vi "UI.vi"() -> (3 "Current File":path)   [LabVIEW 2020, in "FrameEditor.lvlib"]
doc: "This template is for the Queued Message Handler design pattern.\n\nThe Event Handling Loop generates messages based on user interface actions.\n\nThe Message Handling Loop processes messages generated by the Event Handling Loop, or by other messages. The messages are string values, so new messages can be added easily to the Message Cases case structure in the Message Handling Loop. Each message cluster can also provide an optional value for Message Data, which is a variant that can be converted to whatever message-specific data is required."
uses:
  FrameEditor.lvlib
  support/Message Queue/Message Queue.lvlib
  <vilib>/Utility/error.llb/Error Cluster From Error Code.vi
  support/User Event - Stop/User Event - Stop.lvlib
  support/Message Queue/Enqueue Message (Single).vi
  <vilib>/ErrorRing/Error Ring.xnode
  controls/UI Data.ctl
  Azdo/emea-aim-664-instrument-driver-1204/src/AIM664LV.lvlib
  controls/frame_record_type.ctl
  Azdo/emea-aim-664-instrument-driver-1204/src/_controls/queue_header_generic.ctl
  controls/frame_file_entry.ctl
  Azdo/emea-aim-664-instrument-driver-1204/src/_controls/queue_data_full.ctl
panel:
  in  "FrameID":string
  in  "Payload size":u32
  in  "Data":u8[](array[numeric])=[10] format="%.0x"
  in  "Frame Configuration":T1={"domainID"=1, "sideID"=1, "locationID"=1, "interfaceID"=1, "partitionID"=1} {"interfaceID" format="%.0b"}
  in  "VL Id":u16=60
  in  "UDPdstPort":u16=1
  in  "UDPsrcPort":u16=1
  in  "HeaderInfo":T2={"InterFrameGap"=0, "PacketGroupWaitTime"=10000, "PayloadBufferMode"=0, "PayloadGenerationMode"=0, "PreambleCount"=7, "Skew"=0, "NetSelect"=4, "FrameStartMode"=1, "PhysErrorInjection"=0, "SequenceNumberInit"=65535, "SequenceNumberOffset"=65535} {"NetSelect" items=["FDX_TX_FRAME_DLY_A"=0, "FDX_TX_FRAME_DLY_B"=1, "FDX_TX_FRAME_BOTH "=3, "FDX_TX_FRAME_ONLY_A"=4, "FDX_TX_FRAME_ONLY_B "=5]; "FrameStartMode" items=["FDX_TX_FRAME_START_IFG", "FDX_TX_FRAME_START_PGWT", "FDX_TX_FRAME_START_TRG"]; "PhysErrorInjection" items=["FDX_TX_FRAME_ERR_OFF"=0, "FDX_TX_FRAME_ERR_CRC"=1, "FDX_TX_FRAME_ERR_ALI"=2, "FDX_TX_FRAME_ERR_PRE"=4, "FDX_TX_FRAME_ERR_PHY"=8]; "SequenceNumberInit" items=["FDX_TX_FRAME_SEQ_INIT_AUTO"=65535]; "SequenceNumberOffset" items=["FDX_TX_FRAME_SEQ_OFFS_AUTO "=65535]; "PayloadGenerationMode" items=["FDX_TX_FRAME_PGM_USER"=0, "FDX_TX_FRAME_PGM_IP_PART"=1, "FDX_TX_FRAME_PGM_IP_FULL"=2, "FDX_TX_FRAME_PGM_IP_PART_TT"=10, "FDX_TX_FRAME_PGM_IP_FULL_TT"=20]; "PayloadBufferMode" items=["FDX_TX_FRAME_PBM_STD", "FDX_TX_FRAME_PBM_MAC", "FDX_TX_FRAME_PBM_UDP"]}
  in  "Load":bool
  in  "Save":bool
  in  "Frames":i32(listbox)
  out "Display <Replace Me>":string
  in  "Remove":bool
  in  "Add":bool
  in  "Exit":bool
  # "add new"
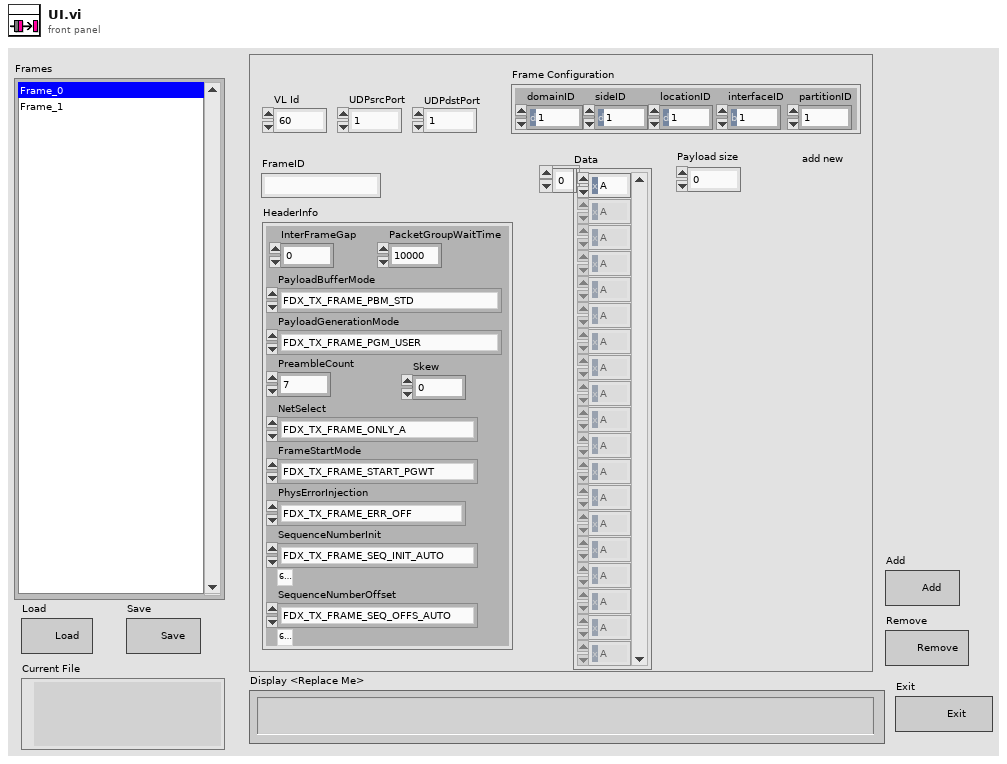
[diagram p1: front panel]
types:
  T1 = typedef "AIM664LV.lvlib/queue_data_full.ctl" = cluster{"domainID":u8, "sideID":u8, "locationID":u8, "interfaceID":u8, "partitionID":u8}
  T2 = typedef "AIM664LV.lvlib/queue_header_generic.ctl" = cluster{"InterFrameGap":u32, "PacketGroupWaitTime":u32, "PayloadBufferMode":u8, "PayloadGenerationMode":u8, "PreambleCount":u8, "Skew":u32, "NetSelect":u8, "FrameStartMode":u8, "PhysErrorInjection":u32, "SequenceNumberInit":u16, "SequenceNumberOffset":u16}
  T3 = typedef "FrameEditor.lvlib/frame_record_type.ctl" = cluster{"HeaderInfo":T2, "Data":u8[]}
  T4 = typedef "FrameEditor.lvlib/UI Data.ctl" = cluster{"Boolean <Replace Me>":bool, "String <Replace Me>":string, "Numeric <Replace Me>":dbl, "Add":refnum<vi>, "Remove":refnum<vi>, "Data Display Ref":refnum<vi>, "Exit Button Ref":refnum<vi>, "Load":refnum<vi>, "Save":refnum<vi>}
  T5 = typedef "FrameEditor.lvlib/Message Queue.lvlib/All Message Queues.ctl" = cluster{"UI":refnum<queue>}
  T6 = typedef "FrameEditor.lvlib/frame_file_entry.ctl" = cluster{"key":string, "value":T3}
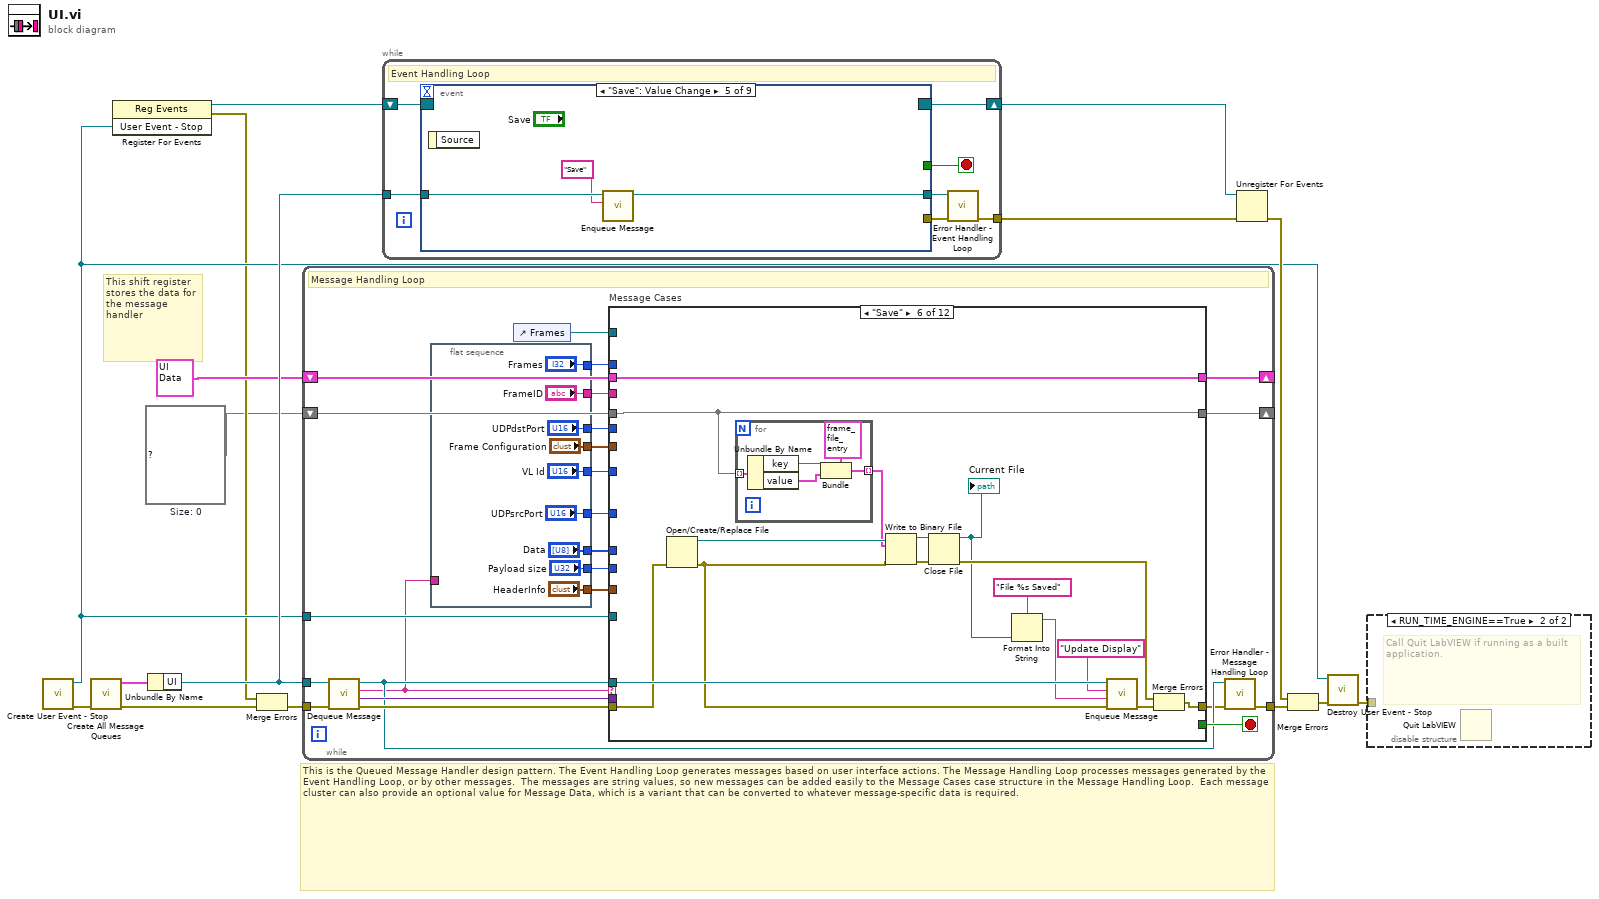
[diagram p0: block diagram]
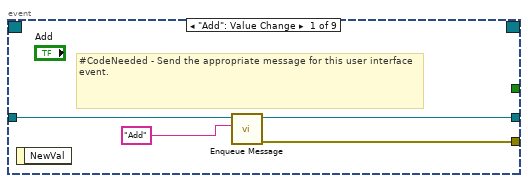
[diagram p3: hidden frame]
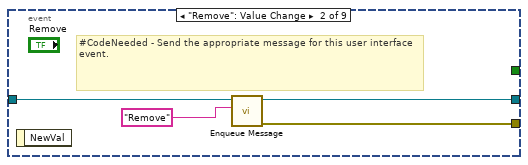
[diagram p4: hidden frame]
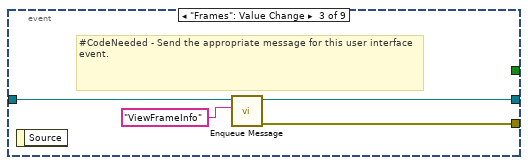
[diagram p5: hidden frame]
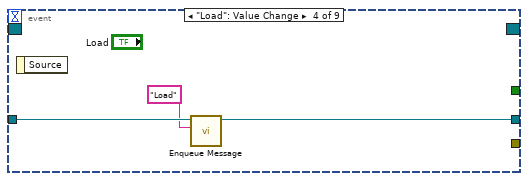
[diagram p6: hidden frame]
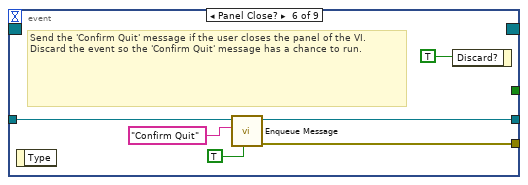
[diagram p7: hidden frame]
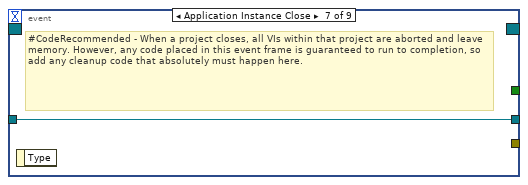
[diagram p8: hidden frame]
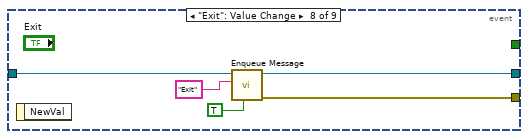
[diagram p9: hidden frame]
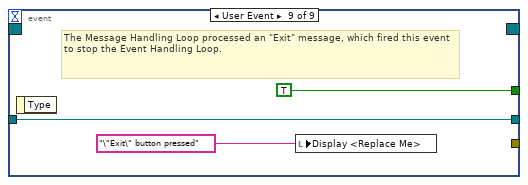
[diagram p10: hidden frame]
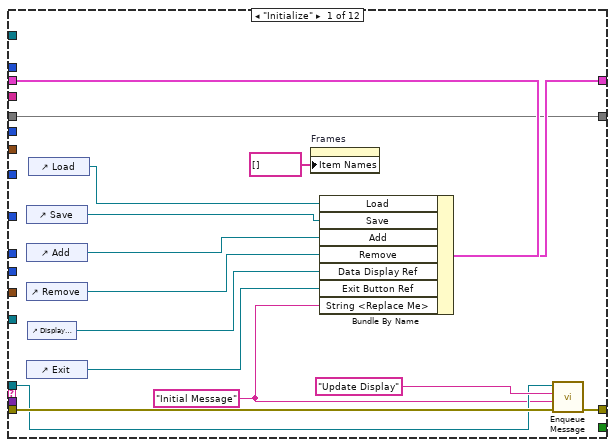
[diagram p11: hidden frame]
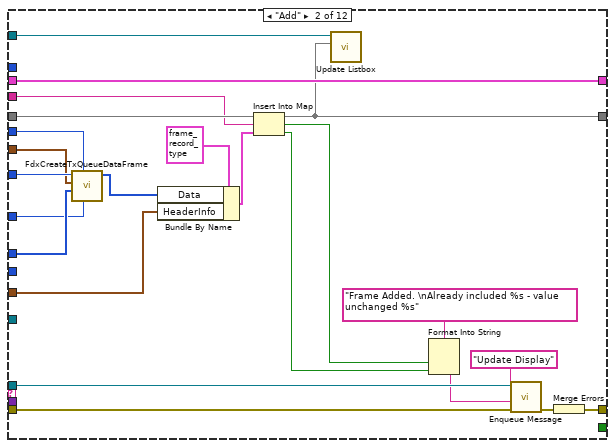
[diagram p12: hidden frame]
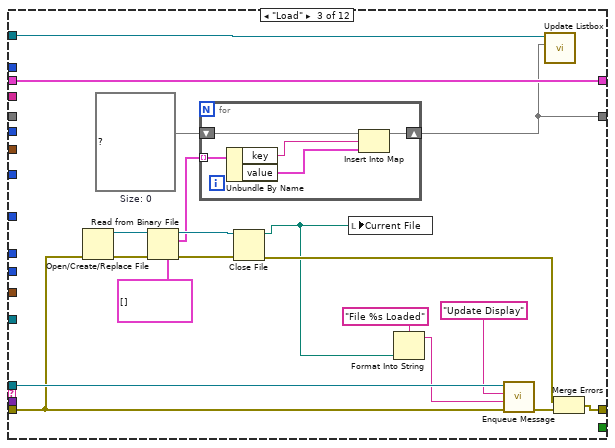
[diagram p13: hidden frame]
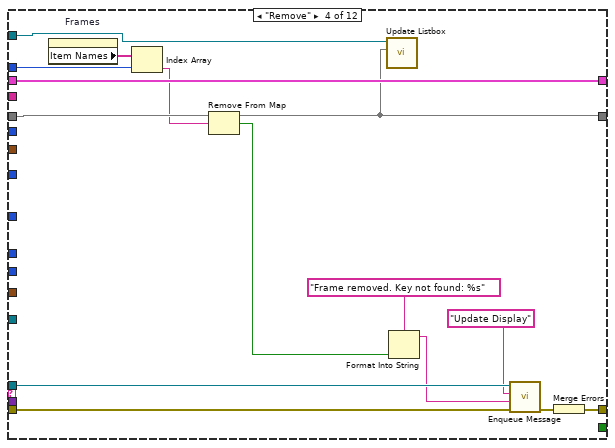
[diagram p14: hidden frame]
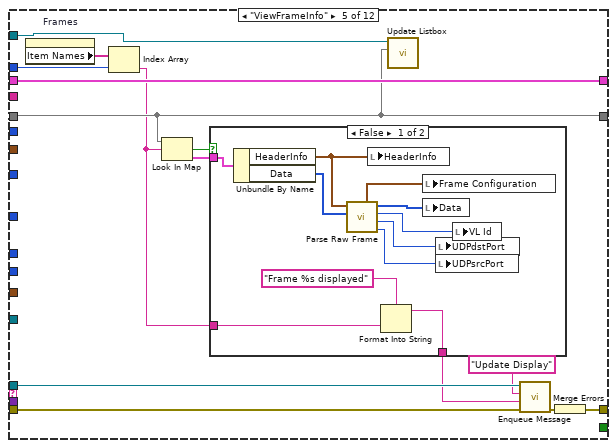
[diagram p15: hidden frame]
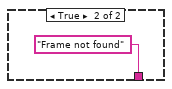
[diagram p16: hidden frame]
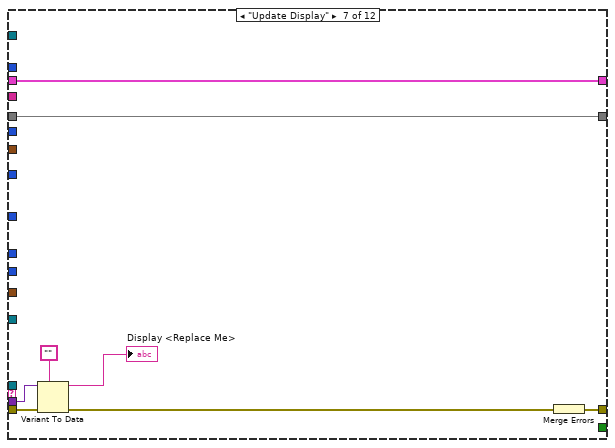
[diagram p17: hidden frame]
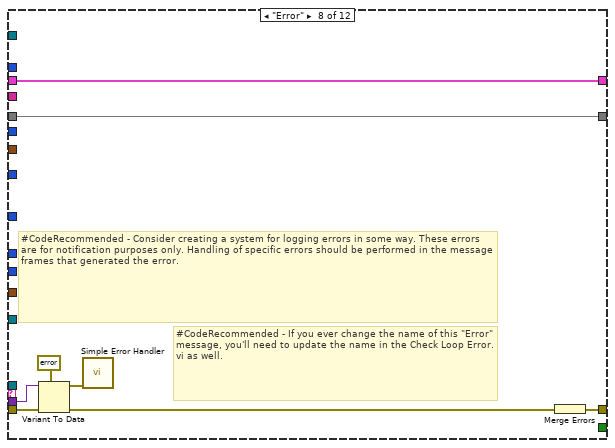
[diagram p18: hidden frame]
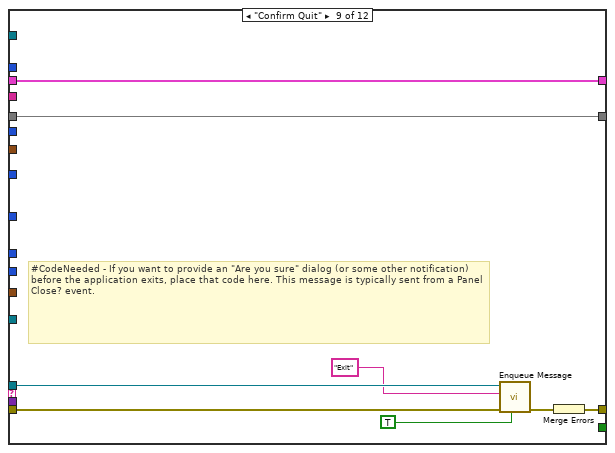
[diagram p19: hidden frame]
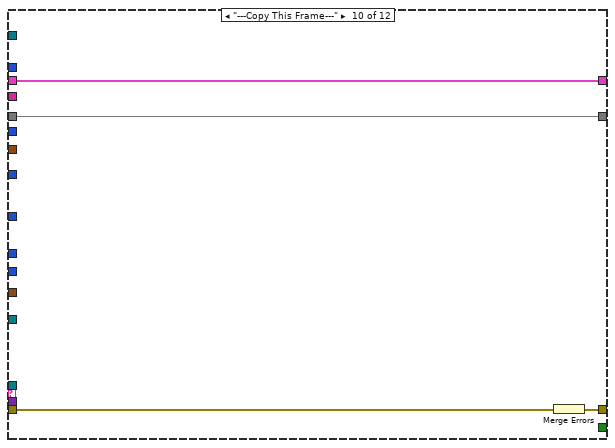
[diagram p20: hidden frame]
diagram:
  w1 = map{string, T3} {}  # Size: 0
  # "This is the Queued Message Handler design pattern. The Event Handling Loop generates messages based on user interface actions. The Message Handling Loop processes messages generated by the Event Handling Loop, or by other messages.  The messages are string values, so new messages can be added easily to the Message Cases case structure in the Message Handling Loop.  Each message cluster can also provide an optional value for Message Data, which is a variant that can be converted to whatever message-specific data is required."
  # "This shift register stores the data for the message handler"
  n1 = call "Create User Event - Stop.vi"() -> ("error out"=w12:errorcluster, "User Event - Stop"=w4:refnum<user-event>)  [unwired: 10 in]
  n2 = call "Create All Message Queues.vi"("error in (no error)"=w12) -> ("error out"=w16:errorcluster, "Message Queues out"=w15:T5)  [unwired: 9 in]
  n3 = register-events(w4) -> (reference out=w5:refnum<event-registration>, error out=w2:errorcluster)  [unwired: 2 in]
  n4 = Unbundle By Name(w15) -> ("UI"=w13:refnum<queue>)
  n5 = Merge Errors(w2, w16) -> (w3:errorcluster)
  n6 = while {
    tunnel: w13 -> [w33]
    shift-right: [w39] -> _
    shift-left: T4 {"Boolean <Replace Me>"=FALSE, "String <Replace Me>"="", "Numeric <Replace Me>"=0.0, "Add"=refnum, "Remove"=refnum, "Data Display Ref"=refnum, "Exit Button Ref"=refnum, "Load"=refnum, "Save"=refnum} ("Data Cluster") -> [w40]
    tunnel: w4 -> [w37]
    tunnel: w3 -> [w36]
    tunnel: [w31] -> w14
    shift-right: [w20] -> _
    shift-left: w1 -> [w22]
    stop <- w38 stop-if-true
    # "Message Handling Loop"
    n7 = call "Dequeue Message.vi"("error in (no error)"=w36, "Message Queue"=w33) -> ("error out"=w35:errorcluster, "Message Data"=w34:variant, "Message"=w17:string, "dup Message Queue"=w32:refnum<queue>)  [unwired: 6 in]
    n8 = flat-sequence {
      tunnel: ["Payload size"] -> w29
      tunnel: ["Frame Configuration"] -> w28
      tunnel: ["VL Id"] -> w27
      tunnel: ["UDPsrcPort"] -> w26
      tunnel: ["UDPdstPort"] -> w25
      tunnel: ["Data"] -> w24
      tunnel: ["HeaderInfo"] -> w23
      tunnel: ["FrameID"] -> w21
      tunnel: ["Frames"] -> w19
      tunnel: w17 -> [_]
      frame #0 {
      }
    }
    n9 = control-ref of="Frames"() -> (w18:refnum<vi>)
    n10 = case "Message Cases" shown="\"Save\"" w17 {
      selector: w17 -> [_ _ _ _ _ _ _ _ _ _ _ w215]
      tunnel: w32 -> [w55 w83 w103 w122 w136 w165 _ _ w193 _ w213 _]
      tunnel: w35 -> [w63 w85 w100 w124 w138 w163 w179 w189 w197 w201 w206 _]
      tunnel: [w64 w86 w105 w125 w139 w167 w180 w183 w195 w199 w209 w216] -> w30
      tunnel: w40 -> [w62 w87 w106 w126 w140 w168 w181 w188 w196 w200 w212 w217]
      tunnel: [w61 w87 w106 w126 w140 w168 w181 w188 w196 w200 w212 w217] -> w39
      tunnel: [_ _ _ _ _ _ _ _ _ _ TRUE _] -> w38
      tunnel: w34 -> [_ _ _ _ _ _ w178 w187 _ _ w203 _]
      tunnel: w37 -> [_ _ _ _ _ _ _ _ _ _ w208 _]
      tunnel: w29 -> [_ _ _ _ _ _ _ _ _ _ _ _]
      tunnel: w28 -> [_ w80 _ _ _ _ _ _ _ _ _ _]
      tunnel: w27 -> [_ w81 _ _ _ _ _ _ _ _ _ _]
      tunnel: w26 -> [_ w77 _ _ _ _ _ _ _ _ _ _]
      tunnel: w25 -> [_ w79 _ _ _ _ _ _ _ _ _ _]
      tunnel: w24 -> [_ w78 _ _ _ _ _ _ _ _ _ _]
      tunnel: w23 -> [_ w72 _ _ _ _ _ _ _ _ _ _]
      tunnel: w22 -> [w51 w76 _ w118 w132 w162 w174 w182 w190 w198 w202 w214]
      tunnel: w21 -> [_ w75 _ _ _ _ _ _ _ _ _ _]
      tunnel: [w51 w69 w91 w115 w132 w162 w174 w182 w190 w198 w202 w214] -> w20
      tunnel: w19 -> [_ _ _ w119 w134 _ _ _ _ _ _ _]
      tunnel: w18 -> [_ w70 w101 w116 w133 _ _ _ _ _ _ _]
      frame "Initialize" {
        w54 = "Initial Message" ("Initial Message")
        # "Initialize - All initialization work should take place in this message, since other loops can potentially enqueue messages that execute immediately after this one."
        n11 = control-ref of="Save"() -> (w52:refnum<vi>)
        n12 = control-ref of="Add"() -> (w60:refnum<vi>)
        n13 = control-ref of="Remove"() -> (w59:refnum<vi>)
        n14 = control-ref of="Exit"() -> (w57:refnum<vi>)
        n15 = control-ref of="Display <Replace Me>"() -> (w58:refnum<vi>)
        n16 = control-ref of="Load"() -> (w53:refnum<vi>)
        n17 = property on="Frames" class="LstBox (strict)"("Item Names"=string[] []) -> ()  [unwired: 2 in, 2 out]
        n18 = Bundle By Name(cluster=w62, "Load"=w53, "Save"=w52, "Add"=w60, "Remove"=w59, "Data Display Ref"=w58, "Exit Button Ref"=w57, "String <Replace Me>"=w54) -> (w61:T4)
        n19 = call-poly "Enqueue Message.vi"("error in (no error)"=w63, "Message Data"=w54, "Message"="Update Display", "Message Queue"=w55) -> ("error out"=w64:errorcluster)  [unwired: 6 in, 1 out]
      }
      frame "Add" {
        # "Something - Replace this message with functionality for your own application."
        n20 = call "FdxCreateTxQueueDataFrame.vi"("UDPsrcPort"=w77, "UDPdstPort"=w79, "Payload"=w78, "afdx configuration"=w80, "VL Id"=w81) -> ("Frame"=w71:u8[])  [unwired: 4 in, 2 out]
        n21 = Bundle By Name(cluster=T3 {"HeaderInfo"={"InterFrameGap"=0, "PacketGroupWaitTime"=10000, "PayloadBufferMode"=0, "PayloadGenerationMode"=0, "PreambleCount"=7, "Skew"=0, "NetSelect"=4, "FrameStartMode"=1, "PhysErrorInjection"=0, "SequenceNumberInit"=65535, "SequenceNumberOffset"=65535}, "Data"=[10]}, "Data"=w71, "HeaderInfo"=w72) -> (w73:T3)
        n22 = Insert Into Map(map in=w76, key=w75, value=w73) -> (map out=w69:map{string, T3}, key already included?=w66:bool, value unchanged?=w65:bool)
        n23 = call "Update Listbox.vi"("frame map"=w69, "ListBox ref"=w70) -> ()  [unwired: 10 in]
        n24 = Format Into String(format string="Frame Added. \nAlready included %s - value unchanged %s", w66, w65) -> (resulting string=w67:string)  [unwired: 2 in, 1 out]
        n25 = call-poly "Enqueue Message.vi"("error in (no error)"=w85, "Message Data"=w67, "Message"="Update Display", "Message Queue"=w83) -> ("error out"=w84:errorcluster)  [unwired: 6 in, 1 out]
        n26 = Merge Errors(w84) -> (w86:errorcluster)
      }
      frame "Load" {
        w93 = map{string, T3} {}  # Size: 0
        # "Something - Replace this message with functionality for your own application."
        n27 = Open/Create/Replace File(error in=w100) -> (refnum out=w95:refnum<file>, error out=w99:errorcluster)  [unwired: 5 in, 1 out]
        n28 = Read from Binary File(5:T6[] [] ("cluster"), 8:w99, 11:w95) -> (0:w98:errorcluster, 2:w92:T6[], 3:w96:refnum<file>)  [unwired: 3 in, 1 out]
        n29 = for {
          shift-right: [w110] -> w91
          shift-left: w93 -> [w111]
          tunnel: w92 -> [w109] mode=indexing
          n30 = Unbundle By Name(w109) -> ("key"=w108:string, "value"=w107:T3)
          n31 = Insert Into Map(map in=w111, key=w108, value=w107) -> (map out=w110:map{string, T3})  [unwired: 2 out]
        }
        n32 = Close File(refnum=w96, error in=w98) -> (path=w88:path, error out=w97:errorcluster)
        n33 = local write "Current File"(w88) -> ()
        n34 = Format Into String(format string="File %s Loaded", w88) -> (resulting string=w89:string)  [unwired: 2 in, 1 out]
        n35 = call-poly "Enqueue Message.vi"("error in (no error)"=w100, "Message Data"=w89, "Message"="Update Display", "Message Queue"=w103) -> ("error out"=w104:errorcluster)  [unwired: 6 in, 1 out]
        n36 = call "Update Listbox.vi"("frame map"=w91, "ListBox ref"=w101) -> ()  [unwired: 10 in]
        n37 = Merge Errors(w97, w104) -> (w105:errorcluster)
      }
      frame "Remove" {
        # "Something Else - Replace this message with functionality for your own application."
        n38 = property on="Frames" class="LstBox (strict)"() -> ("Item Names"=w120:string[])  [unwired: 2 in, 2 out]
        n39 = Index Array(array=w120, index=w119) -> (element=w117:string)
        n40 = Remove From Map(10:w117, 11:w118) -> (2:w112:bool, 3:w115:map{string, T3})  [unwired: 1 out]
        n41 = call "Update Listbox.vi"("frame map"=w115, "ListBox ref"=w116) -> ()  [unwired: 10 in]
        n42 = Format Into String(format string="Frame removed. Key not found: %s", w112) -> (resulting string=w113:string)  [unwired: 2 in, 1 out]
        n43 = call-poly "Enqueue Message.vi"("error in (no error)"=w124, "Message Data"=w113, "Message"="Update Display", "Message Queue"=w122) -> ("error out"=w123:errorcluster)  [unwired: 6 in, 1 out]
        n44 = Merge Errors(w123) -> (w125:errorcluster)
      }
      frame "ViewFrameInfo" {
        # "Something Else - Replace this message with functionality for your own application."
        n45 = property on="Frames" class="LstBox (strict)"() -> ("Item Names"=w135:string[])  [unwired: 2 in, 2 out]
        n46 = Index Array(array=w135, index=w134) -> (element=w127:string)
        n47 = Look In Map(map=w132, key=w127) -> (key not found?=w131:bool, value=w130:T3)  [unwired: 1 in]
        n48 = case shown="False" w131 {
          tunnel: w130 -> [w151 _]
          tunnel: [w148 "Frame not found"] -> w128
          tunnel: w127 -> [w149 _]
          frame False {
            n49 = Unbundle By Name(w151) -> ("HeaderInfo"=w147:T2, "Data"=w144:u8[])
            n50 = call "Parse Raw Frame.vi"("Data"=w144, "HeaderInfo"=w147) -> ("UDPsrcPort"=w141:u16, "UDPdstPort"=w142:u16, "VL Id"=w143:u16, "Payload"=w146:u8[], "Frame Configuration"=w145:T1)  [unwired: 5 in]
            n51 = local write "HeaderInfo"(w147) -> ()
            n52 = Format Into String(format string="Frame %s displayed", w149) -> (resulting string=w148:string)  [unwired: 2 in, 1 out]
            n53 = local write "Frame Configuration"(w145) -> ()
            n54 = local write "Data"(w146) -> ()
            n55 = local write "UDPdstPort"(w142) -> ()
            n56 = local write "UDPsrcPort"(w141) -> ()
            n57 = local write "VL Id"(w143) -> ()
          }
          frame True {
          }
        }
        n58 = call "Update Listbox.vi"("frame map"=w132, "ListBox ref"=w133) -> ()  [unwired: 10 in]
        n59 = call-poly "Enqueue Message.vi"("error in (no error)"=w138, "Message Data"=w128, "Message"="Update Display", "Message Queue"=w136) -> ("error out"=w137:errorcluster)  [unwired: 6 in, 1 out]
        n60 = Merge Errors(w137) -> (w139:errorcluster)
      }
      frame "Save" {
        # "Something Else - Replace this message with functionality for your own application."
        n61 = Open/Create/Replace File(error in=w163) -> (refnum out=w161:refnum<file>, error out=w160:errorcluster)  [unwired: 5 in, 1 out]
        n62 = for {
          tunnel: w162 -> [w173] mode=indexing
          tunnel: [w170] -> w156 mode=indexing
          n63 = Unbundle By Name(w173) -> ("key"=w172:string, "value"=w171:T3)
          n64 = Bundle(cluster=T6 {"key"="", "value"={"HeaderInfo"={"InterFrameGap"=0, "PacketGroupWaitTime"=0, "PayloadBufferMode"=0, "PayloadGenerationMode"=0, "PreambleCount"=0, "Skew"=0, "NetSelect"=0, "FrameStartMode"=0, "PhysErrorInjection"=0, "SequenceNumberInit"=0, "SequenceNumberOffset"=0}, "Data"=[]}}, "key"=w172, "value"=w171) -> (w170:T6)
        }
        n65 = Write to Binary File(file (use dialog)=w161, data=w156, error in=w160) -> (refnum out=w158:refnum<file>, error out=w159:errorcluster)  [unwired: 3 in, 1 out]
        n66 = Close File(refnum=w158, error in=w159) -> (path=w153:path, error out=w157:errorcluster)
        "Current File" <- w153
        n67 = Format Into String(format string="File %s Saved", w153) -> (resulting string=w155:string)  [unwired: 2 in, 1 out]
        n68 = call-poly "Enqueue Message.vi"("error in (no error)"=w160, "Message Data"=w155, "Message"="Update Display", "Message Queue"=w165) -> ("error out"=w166:errorcluster)  [unwired: 6 in, 1 out]
        n69 = Merge Errors(w157, w166) -> (w167:errorcluster)
      }
      frame "Update Display" {
        # "Update Display - Convert the message data to a string to display in the Data Display indicator."
        n70 = Variant To Data(error in=w179, type="", Variant=w178) -> (data=→"Display <Replace Me>":string, error out=w176:errorcluster)
        n71 = Merge Errors(w176) -> (w180:errorcluster)
      }
      frame "Error" {
        # "#CodeRecommended - If you ever change the name of this \"Error\" message, you'll need to update the name in the Check Loop Error.vi as well."
        # "#CodeRecommended - Consider creating a system for logging errors in some way. These errors are for notification purposes only. Handling of specific errors should be performed in the message frames that generated the error."
        # "Error - Display an error dialog. This message is sent by the \"Error Handler\" VIs at the end of other loops in this application."
        n72 = Variant To Data(error in=w189, type=errorcluster {"status"=FALSE, "code"=0, "source"=""} ("error constant"), Variant=w187) -> (data=w185:errorcluster, error out=w184:errorcluster)
        n73 = call <vilib>:"Simple Error Handler.vi"("error in (no error)"=w185) -> ()  [unwired: 4 in, 5 out]
        n74 = Merge Errors(w184) -> (w183:errorcluster)
      }
      frame "Confirm Quit" {
        # "#CodeNeeded - If you want to provide an \"Are you sure\" dialog (or some other notification) before the application exits, place that code here. This message is typically sent from a Panel Close? event."
        # "Confirm Quit - Message that can confirm whether or not the user wants to exit the application."
        n75 = call-poly "Enqueue Message.vi"("Priority Message? (F)"=TRUE, "error in (no error)"=w197, "Message"="Exit", "Message Queue"=w193) -> ("error out"=w194:errorcluster)  [unwired: 6 in, 1 out]
        n76 = Merge Errors(w194) -> (w195:errorcluster)
      }
      frame "---Copy This Frame---" {
        # "Duplicate this frame when creating new messages.  Change this comment in the duplicated frame to describe this message."
        n77 = Merge Errors(w201) -> (w199:errorcluster)
      }
      frame "Exit" {
        # "Stop the VI"
        # "Release the message queue reference"
        # "#CodeNeeded - Add any required cleanup code here. Note that if 'Exit' was called as a result of an error, an error dialog will be displayed. Add any custom error handling for an 'Exit' condition here as well."
        # "Exit - Exit the application."
        n78 = Variant To Data(type=errorcluster {"status"=FALSE, "code"=0, "source"=""} ("error constant"), Variant=w203) -> (data=w204:errorcluster)  [unwired: 1 in, 1 out]
        n79 = call <vilib>:"Simple Error Handler.vi"("error in (no error)"=w204) -> ()  [unwired: 4 in, 5 out]
        n80 = call "Fire User Event - Stop.vi"("User Event - Stop"=w208) -> ("error out"=w207:errorcluster)  [unwired: 10 in]
        n81 = Release Queue(queue=w213, error in (no error)=w206) -> (error out=w210:errorcluster)  [unwired: 1 in, 2 out]
        n82 = Merge Errors(w207, w210) -> (w209:errorcluster)
      }
      frame Default {
        # "'Default' case only runs if there is a message that isn't defined in any of the other cases.  Output a programming error."
        n83 = xnode "Error Ring"("parameter 0"=w215) -> ("error out"=w216:errorcluster)
      }
    }
    n84 = call "Error Handler - Message Handling Loop.vi"("error in (no error)"=w30, "Message Queue"=w32) -> ("dup error in"=w31:errorcluster)  [unwired: 8 in, 1 out]
  }
  n85 = while {
    tunnel: w13 -> [w231]
    shift-right: [w229] -> w9
    shift-left: w5 -> [w230]
    tunnel: [w225] -> w6
    stop <- w227 stop-if-true
    # "Event Handling Loop"
    n86 = event shown="[4] \"Save\": Value Change" {
      selector: w230 -> [_ _ _ _ _ _ _ _ _]
      dyn-events: [_ _ _ _ _ _ _ _ _] -> w229
      timeout: _ -> [_ _ _ _ _ _ _ _ _]
      tunnel: [_ _ _ _ _ _ _ _ TRUE ("Discard?")] -> w227
      tunnel: w231 -> [w235 w239 w243 w246 w249 w254 w256 w261 w264]
      tunnel: [w232 w236 w240 _ _ w253 _ w260 _] -> w228
      tunnel: [w234 w238 w242 w245 w248 w252 w256 w259 w264] -> w226
      event "Add": Value Change {
        # "#CodeNeeded - Send the appropriate message for this user interface event."
        n87 = event-data() -> ()  [unwired: 1 in, 1 out]
        n88 = call-poly "Enqueue Message.vi"("Message"="Add", "Message Queue"=w235) -> ("error out"=w232:errorcluster, "dup Message Queue"=w234:refnum<queue>)  [unwired: 8 in]
      }
      event "Remove": Value Change {
        # "#CodeNeeded - Send the appropriate message for this user interface event."
        n89 = event-data() -> ()  [unwired: 1 in, 1 out]
        n90 = call-poly "Enqueue Message.vi"("Message"="Remove", "Message Queue"=w239) -> ("error out"=w236:errorcluster, "dup Message Queue"=w238:refnum<queue>)  [unwired: 8 in]
      }
      event "Frames": Value Change {
        # "#CodeNeeded - Send the appropriate message for this user interface event."
        n91 = event-data() -> ()  [unwired: 1 in, 1 out]
        n92 = call-poly "Enqueue Message.vi"("Message"="ViewFrameInfo", "Message Queue"=w243) -> ("error out"=w240:errorcluster, "dup Message Queue"=w242:refnum<queue>)  [unwired: 8 in]
      }
      event "Load": Value Change {
        n93 = event-data() -> ()  [unwired: 1 in, 1 out]
        n94 = call-poly "Enqueue Message.vi"("Message"="Load", "Message Queue"=w246) -> ("dup Message Queue"=w245:refnum<queue>)  [unwired: 8 in, 1 out]
      }
      event "Save": Value Change {
        n95 = event-data() -> ()  [unwired: 1 in, 1 out]
        n96 = call-poly "Enqueue Message.vi"("Message"="Save", "Message Queue"=w249) -> ("dup Message Queue"=w248:refnum<queue>)  [unwired: 8 in, 1 out]
      }
      event Panel Close? {
        # "Send the 'Confirm Quit' message if the user closes the panel of the VI. Discard the event so the 'Confirm Quit' message has a chance to run."
        n97 = event-data() -> ()  [unwired: 1 in, 1 out]
        n98 = call-poly "Enqueue Message.vi"("Priority Message? (F)"=TRUE, "Message"="Confirm Quit", "Message Queue"=w254) -> ("error out"=w253:errorcluster, "dup Message Queue"=w252:refnum<queue>)  [unwired: 7 in]
        n99 = event-data("Discard?"=TRUE) -> ()  [unwired: 1 in, 1 out]
      }
      event Application Instance Close {
        # "#CodeRecommended - When a project closes, all VIs within that project are aborted and leave memory. However, any code placed in this event frame is guaranteed to run to completion, so add any cleanup code that absolutely must happen here."
        n100 = event-data() -> ()  [unwired: 1 in, 1 out]
      }
      event "Exit": Value Change {
        n101 = event-data() -> ()  [unwired: 1 in, 1 out]
        n102 = call-poly "Enqueue Message.vi"("Priority Message? (F)"=TRUE, "Message"="Exit", "Message Queue"=w261) -> ("error out"=w260:errorcluster, "dup Message Queue"=w259:refnum<queue>)  [unwired: 7 in]
      }
      event User Event {
        # "The Message Handling Loop processed an \"Exit\" message, which fired this event to stop the Event Handling Loop."
        n103 = event-data() -> ()  [unwired: 1 in, 1 out]
        n104 = local write "Display <Replace Me>"("\"Exit\" button pressed" ("VI Stopped")) -> ()
      }
    }
    n105 = call "Error Handler - Event Handling Loop.vi"("error in (no error)"=w228, "Message Queue"=w226) -> ("dup error in"=w225:errorcluster)  [unwired: 8 in, 1 out]
  }
  n106 = Unregister For Events(event registration refnum=w9, error in=w6) -> (error out=w10:errorcluster)
  n107 = Merge Errors(w10, w14) -> (w11:errorcluster)
  n108 = call "Destroy User Event - Stop.vi"("error in (no error)"=w11, "User Event - Stop"=w4) -> ("error out"=w7:errorcluster)  [unwired: 9 in]
  n109 = disable-structure shown="RUN_TIME_ENGINE==True" {
    disable-tunnel: w7 -> [_ _]
    frame condition #0 (active) {
    }
    frame condition #1 {
      # "Call Quit LabVIEW if running as a built application."
      n110 = Quit LabVIEW() -> ()  [unwired: 1 in]
    }
  }
